vi "Demo-GetDXF.vi"() -> ()   [LabVIEW 2019]
uses:
  <userlib>/IoT Devices/_subVIs/HTTPComm.ctl
  <userlib>/Onshape/_SubVI/z did wid and eid.vi
panel:
  out "DXF Text":string
  out "Comm":T1
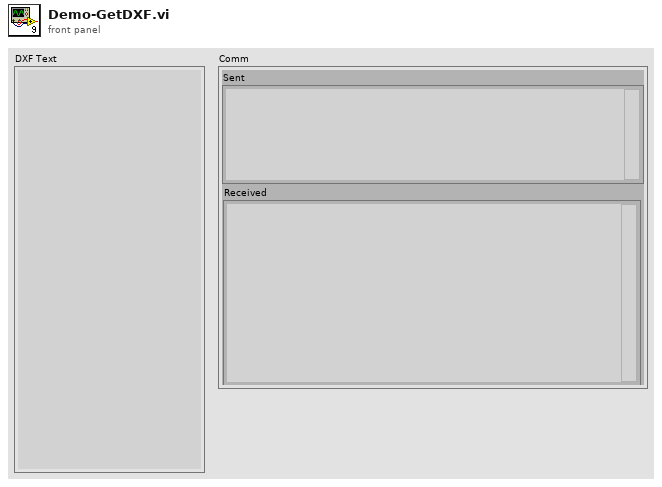
[diagram p1: front panel]
types:
  T1 = typedef "HTTPComm.ctl" = cluster{"url":string, "sent headers":string, "sent body":string, "headers":string, "body":string, "Sent":string, "Received":string}
  T2 = typedef "Cluster.ctl" = cluster{"Date":string, "On-Nonce":string, "eid":string, "wid":string, "did":string, "name":string, "method":string, "Accept":string, "User-Agent":string, "Content-Type":string, "stack":string, "headers":string[], "payload":string, "addition":string, "path":string, "Authorization":string, "secret_key":string, "access_key":string}
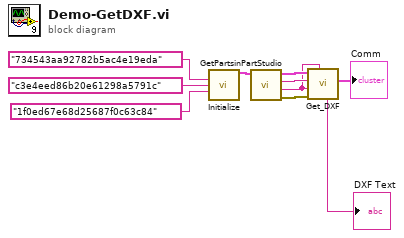
[diagram p0: block diagram]
diagram:
  n1 = call-poly <userlib>:"Initialize.vi"("did"="734543aa92782b5ac4e19eda", "wid"="c3e4eed86b20e61298a5791c", "eid"="1f0ed67e68d25687f0c63c84") -> ("Device Out"=w10:T2)  [unwired: 11 in, 1 out]
  n2 = call "GetPartsinPartStudio.vi"("Device In"=w10) -> ("error out"=w1:errorcluster, "id"=w2:string, "documentMicroversion"=w3:string, "Device Out"=w4:T2)  [unwired: 7 in]
  n3 = call "Get_DXF.vi"("Save as"=w2, "error in"=w1, "Part Id"=w2, "microversion"=w3, "Device In"=w4) -> ("Comm"=→"Comm":T1, "DXF Text"=→"DXF Text":string)  [unwired: 3 in, 2 out]
